vi "test Digital Pattern Output.vi"(8 "error in (no error)":errorcluster, 11 "TestCase in":refnum<class "Engine Simulation IO System Tests.lvclass">) -> (0 "error out":errorcluster, 3 "TestCase out":refnum<class "Engine Simulation IO System Tests.lvclass">)   [LabVIEW 2015, in "Engine Simulation IO System Tests.lvclass"]
uses:
  Engine Simulation IO System Tests.lvclass
  Engine Simulation IO System Tests.lvclass/Engine Simulation IO System Tests.ctl
  <vilib>/NI/LVFPGA Adv Session Resources/OpenByNameSubVI.vi
  <vilib>/NI Veristand/Execution/Workspace/NI VeriStand - Set Single Channel Value.vi
  <vilib>/rvi/interface/common/dynamic/niFpgaEscapeDelimiterAndNull.vi
  <vilib>/Utility/error.llb/Error Cluster From Error Code.vi
  <vilib>/rvi/errors/niLvFpgaAdjustHostInterfaceError.vi
  <vilib>/FPGAPlugInAG/Dynamic/niLvFpga_Close_Dynamic.vi
  <vilib>/NI/LVFPGA Adv Session Resources/OpenByName.xnode
  <vilib>/rvi/interface/nirviReadWriteControl/nirviReadWriteControl.xnode
  <vilib>/rvi/interface/nirviCloseFPGA/nirviCloseFPGA.xnode
  <vilib>/addons/_JKI Toolkits/VI Tester/TestCase.llb/TestCase.lvclass
  <vilib>/NI VeriStand/Execution/Workspace/NI_VS Workspace ExecutionAPI.lvlib
  System Explorer/Digital Pattern Find Events Enum.ctl
  System Explorer/Engine Simulation Toolkit System Explorer.lvlib
  NiFpgaLv.dll
  <vilib>/rvi/interface/Simulation/niFpgaSimulationCallBeginRW.vi
  System Explorer/Digital Pattern Add Pulse.ctl
  System Explorer/Digital Pattern Remove Edge.ctl
  System Explorer/Digital Pattern Base.ctl
  System Explorer/Digital Pattern.ctl
  <vilib>/NI/LVFPGA Adv Session Resources/LVFPGAAdvSessionResources.lvlib
panel:
  out "Values":T1(array[cluster])
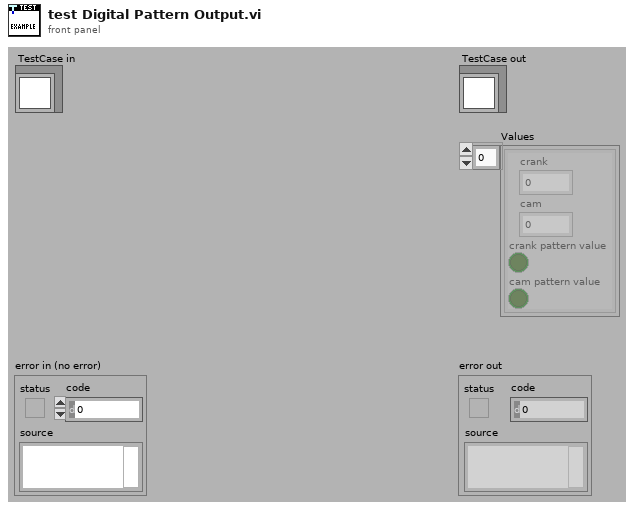
[diagram p1: front panel]
types:
  T1 = cluster{"crank":u16, "cam":u16, "crank pattern value":bool, "cam pattern value":bool}[]
  T2 = typedef "Engine Simulation Toolkit System Explorer.lvlib/Digital Pattern.ctl" = cluster{"Name":string, "Base":T3, "Remove":T4[], "Add":T5[], "FPGA Resource":string}
  T3 = typedef "Engine Simulation Toolkit System Explorer.lvlib/Digital Pattern Base.ctl" = cluster{"Length":dbl, "Teeth":u16, "Width":dbl, "Offset":dbl}
  T4 = typedef "Engine Simulation Toolkit System Explorer.lvlib/Digital Pattern Remove Edge.ctl" = cluster{"Tooth":u16, "Edge":bool}
  T5 = typedef "Engine Simulation Toolkit System Explorer.lvlib/Digital Pattern Add Pulse.ctl" = cluster{"Tooth":u16, "Offset":dbl, "Width":dbl}
  T6 = typedef "Engine Simulation Toolkit System Explorer.lvlib/Digital Pattern Find Events Enum.ctl" = enum16{"Rising Edge", "Falling Edge", "Any Edge", "Center Tooth", "Center Gap"}
  T7 = cluster{"Name":string, "Depth":u32, "Write? (Deprecated:Use Implementation)":bool, "Physical Channel":u32, "Base Address":u32, "Data Width":u32, "Data Type":enum32{"Boolean", "I8", "I16", "I32", "I64", "U8", "U16", "U32", "U64", "FXP", "CustomControl", "SGL"}, "FXP Properties":variant, "Write Window Address":u32, "Implementation":enum16{"niFpgaTargetToHost", "niFpgaHostToTarget", "niFpgaPeerToPeerWriter", "niFpgaPeerToPeerReader", "niCoreTargetToHost", "niCoreHostToTarget"}, "Control Set":u32}[]
  T8 = cluster{"Name":string, "type":variant, "indicator?":bool}[]
  T9 = typedef "NI_VS Workspace ExecutionAPI.lvlib/WorkspaceAPI.ctl" = refnum<k24>
  T10 = typedef "Engine Simulation Toolkit System Explorer.lvlib/Digital Pattern Expanded.ctl" = cluster{"X":dbl[], "Y":dbl[]}
  T11 = cluster{"crank":u16, "cam":u16, "crank pattern value":bool, "cam pattern value":bool}
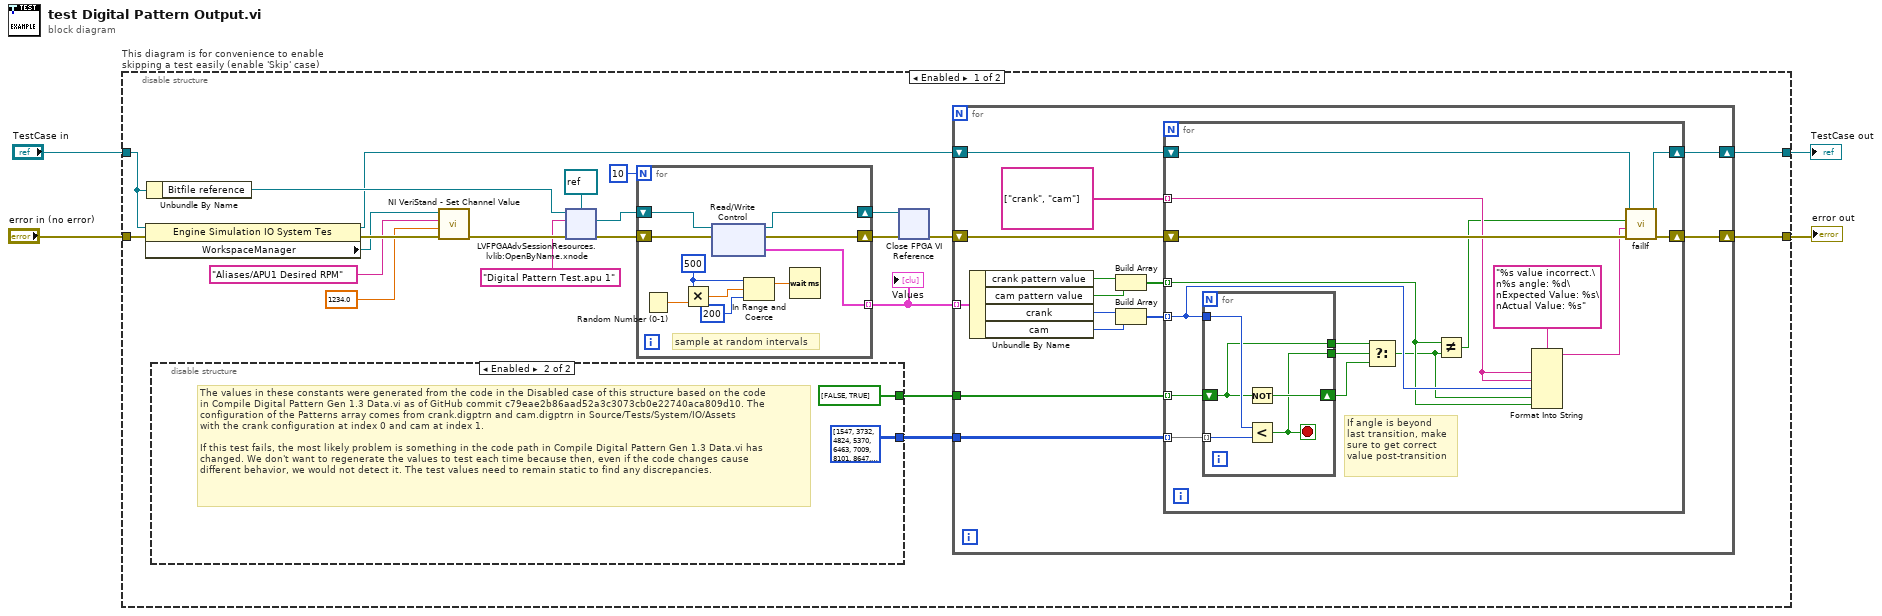
[diagram p0: block diagram]
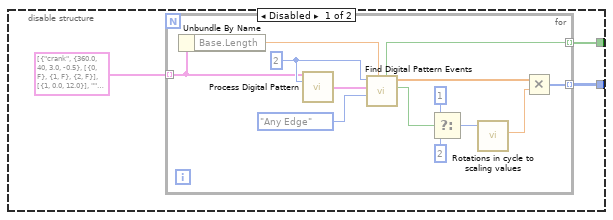
[diagram p2: hidden frame]
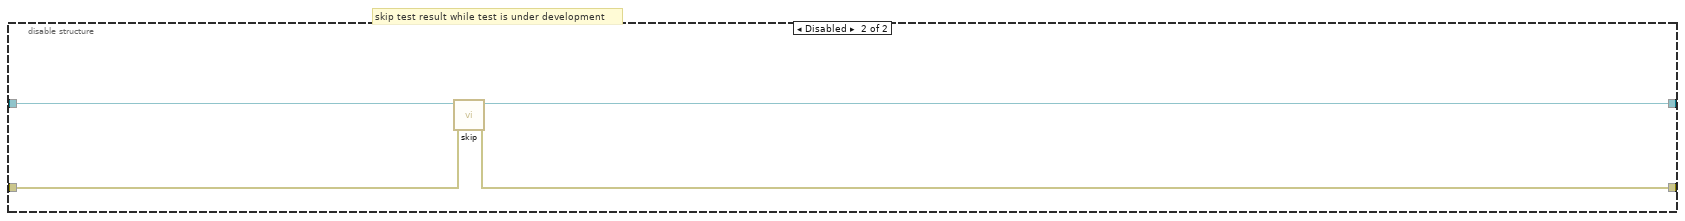
[diagram p3: hidden frame]
diagram:
  n1 = disable-structure "This diagram is for convenience to enable skipping a test easily (enable 'Skip' case)" shown="Enabled" {
    disable-tunnel: "TestCase in" -> [w9 w106]
    disable-tunnel: [w8 w104] -> w1
    disable-tunnel: [w5 w105] -> w3
    disable-tunnel: "error in (no error)" -> [w26 w103]
    frame Enabled {
      n2 = property class="Engine Simulation IO System Tes"(reference=w9, error in=w26) -> (reference out=w7:refnum<class "Engine Simulation IO System Tests.lvclass">, error out=w25:errorcluster, "WorkspaceManager"=w24:T9)
      n3 = Unbundle By Name(w9) -> ("Bitfile reference"=w20:refnum<k20>)
      n4 = disable-structure shown="Enabled" {
        disable-tunnel: [w29 bool[] [FALSE, TRUE] ("First Falling")] -> w11
        disable-tunnel: [w28 u16[][] [[1547, 3732, 4824, 5370, 6463, 7009, 8101, 8647, 9739, 10286, 11378, 11924, 13016, 13562, 14655, 15201, 16293, 16839, 17931, 18478, 19570, 20116, 21208, 21754, 22847, 23393, 24485, 25031, 26123, 26670, 27762, 28308, 29400, 29946, 31039, 31585, 32677, 33223, 34315, 34862, 35954, 36500, 37592, 38138, 39231, 39777, 40869, 41415, 42507, 43054, 44146, 44692, 45784, 46330, 47423, 47969, 49061, 49607, 50699, 51246, 52338, 52884, 53976, 54522, 55615, 56161, 57253, 57799, 58891, 59438, 60530, 61076, 62168, 62714, 63807, 64353], [4506, 13062, 17613, 26169, 30720, 39276, 43827, 52383, 56934, 65490, 0, 0, 0, 0, 0, 0, 0, 0, 0, 0, 0, 0, 0, 0, 0, 0, 0, 0, 0, 0, 0, 0, 0, 0, 0, 0, 0, 0, 0, 0, 0, 0, 0, 0, 0, 0, 0, 0, 0, 0, 0, 0, 0, 0, 0, 0, 0, 0, 0, 0, 0, 0, 0, 0, 0, 0, 0, 0, 0, 0, 0, 0, 0, 0, 0, 0]] ("Position LUT")] -> w10
        frame Disabled {
          n5 = for {
            tunnel: T2[] [{"Name"="crank", "Base"={"Length"=360.0, "Teeth"=40, "Width"=3.0, "Offset"=-0.5}, "Remove"=[{"Tooth"=0, "Edge"=FALSE}, {"Tooth"=1, "Edge"=FALSE}, {"Tooth"=2, "Edge"=FALSE}], "Add"=[{"Tooth"=1, "Offset"=0.0, "Width"=12.0}], "FPGA Resource"=""}, {"Name"="cam", "Base"={"Length"=720.0, "Teeth"=5, "Width"=50.0, "Offset"=-0.5}, "Remove"=[], "Add"=[], "FPGA Resource"=""}] ("Patterns") -> [w39] mode=indexing
            tunnel: [w36] -> w28 mode=indexing
            tunnel: [w30] -> w29 mode=indexing
            w41 = u16 2 ("Rotations")
            n6 = Unbundle By Name(w39) -> ("Base.Length"=w31:dbl)
            n7 = call "Process Digital Pattern.vi"("EPT Pattern"=w39, "Rotations"=w41) -> ("Final"=w42:T10)  [unwired: 7 in, 6 out]
            n8 = call "Find Digital Pattern Events.vi"("Base.length"=w31, "Event"=Digital_Pattern_Find_Events_Enum."Any Edge", "Pattern"=w42, "Rotations"=w41) -> ("crank angle"=w33:bool, "Locations"=w38:dbl[], "first falling"=w30:bool)  [unwired: 5 in]
            n9 = Select(t=u16 1 ("Rotations"), s=w33, f=u16 2 ("Rotations")) -> (s? t:f=w32:u16)
            n10 = call "Rotations in cycle to scaling values.vi"("rotations in a cycle"=w32) -> ("angle to u16 scale factor"=w37:dbl)  [unwired: 8 in, 2 out]
            n11 = Multiply(x=w38, y=w37) -> (x*y=w36:u16[])
          }
        }
        frame Enabled {
          # "The values in these constants were generated from the code in the Disabled case of this structure based on the code\nin Compile Digital Pattern Gen 1.3 Data.vi as of GitHub commit c79eae2b86aad52a3c3073cb0e22740aca809d10. The\nconfiguration of the Patterns array comes from crank.digptrn and cam.digptrn in Source/Tests/System/IO/Assets\nwith the crank configuration at index 0 and cam at index 1.\n\nIf this test fails, the most likely problem is something in the code path in Compile Digital Pattern Gen 1.3 Data.vi has\nchanged. We don't want to regenerate the values to test each time because then, even if the code changes cause\ndifferent behavior, we would not detect it. The test values need to remain static to find any discrepancies."
        }
      }
      n12 = call-poly <vilib>:"NI VeriStand - Set Channel Value.vi"("error in (no error)"=w25, "Value"=1234.0, "Channel"="Aliases/APU1 Desired RPM", "WorkspaceManager in"=w24) -> ("error out"=w21:errorcluster)  [unwired: 6 in, 1 out]
      n13 = xnode "LVFPGAAdvSessionResources.lvlib:OpenByName.xnode"("FPGA VI Reference in"=w20, "Resource name in"="Digital Pattern Test.apu 1", "Single resource reference type in"=refnum<k20> refnum, "Error in"=w21) -> ("Single resource reference out"=w16:refnum<k20>, "Error out"=w17:errorcluster)  [unwired: 1 out]
      n14 = for {
        N: 10 -> [_]
        shift-right: [w88] -> w14
        shift-left: w17 -> [w89]
        shift-right: [w86] -> w13
        shift-left: w16 -> [w87]
        tunnel: [w85] -> w12 mode=indexing
        w83 = u32 500 ("milliseconds to wait")
        # "sample at random intervals"
        n15 = Random Number (0-1)() -> (number: 0 to 1=w84:dbl)
        n16 = Multiply(x=w83, y=w84) -> (x*y=w82:dbl)
        n17 = xnode "Read/Write Control"("FPGA VI Reference In"=w87, "error in"=w89) -> ("FPGA VI Reference Out"=w86:refnum<k20>, "error out"=w88:errorcluster, "Value"=w85:T11)
        n18 = In Range and Coerce(upper limit=w83, x=w82, lower limit=u32 200 ("milliseconds to wait")) -> (coerced(x)=w80:dbl)  [unwired: 1 out]
        n19 = Wait (ms)(milliseconds to wait=w80) -> ()  [unwired: 1 out]
      }
      "Values" <- w12
      n20 = xnode "Close FPGA VI Reference"("FPGA VI Reference In"=w13, "error in"=w14) -> ("error out"=w6:errorcluster)
      n21 = for {
        tunnel: w12 -> [w58] mode=indexing
        tunnel: w11 -> [w57]
        tunnel: w10 -> [w56]
        shift-right: [w51] -> w8
        shift-left: w7 -> [w52]
        shift-right: [w49] -> w5
        shift-left: w6 -> [w50]
        n22 = Unbundle By Name(w58) -> ("crank pattern value"=w48:bool, "cam pattern value"=w47:bool, "crank"=w55:u16, "cam"=w54:u16)
        n23 = Build Array(w48, w47) -> (w46:bool[])
        n24 = Build Array(w55, w54) -> (w53:u16[])
        n25 = for {
          tunnel: w57 -> [w73] mode=indexing
          tunnel: w56 -> [w74] mode=indexing
          tunnel: w53 -> [w64] mode=indexing
          shift-right: [w70] -> w51
          shift-left: w52 -> [w69]
          shift-right: [w71] -> w49
          shift-left: w50 -> [w72]
          tunnel: w46 -> [w63] mode=indexing
          tunnel: string[] ["crank", "cam"] -> [w67] mode=indexing
          # "If angle is beyond\nlast transition, make\nsure to get correct\nvalue post-transition"
          n26 = for {
            tunnel: w74 -> [w78] mode=indexing
            tunnel: w64 -> [w79]
            shift-right: [w77] -> w60
            shift-left: w73 -> [w76]
            tunnel: [w76] -> w61
            tunnel: [w75] -> w62
            stop <- w75 stop-if-true
            n27 = Not(x=w76) -> (.not. x?=w77:bool)
            n28 = Less?(x=w79, y=w78) -> (x < y?=w75:bool)
          }
          n29 = Select(t=w61, s=w62, f=w60) -> (s? t:f=w59:bool)
          n30 = Not Equal?(x=w63, y=w59) -> (x != y?=w66:bool)
          n31 = Format Into String(format string="%s value incorrect.\n%s angle: %d\nExpected Value: %s\nActual Value: %s", w67, w67, w64, w59, w63) -> (resulting string=w65:string)  [unwired: 2 in, 1 out]
          n32 = call-dynamic "failIf.vi"("error in (no error)"=w72, "message (\"\")"=w65, "fail"=w66, "TestCase in"=w69) -> ("error out"=w71:errorcluster, "TestCase out"=w70:refnum<class "Engine Simulation IO System Tests.lvclass">)  [unwired: 6 in]
        }
      }
    }
    frame Disabled {
      # "skip test result while test is under development"
      n33 = call <vilib>:"skip.vi"("error in (no error)"=w103, "TestCase in"=w106) -> ("error out"=w105:errorcluster, "TestCase out"=w104:refnum<class "Engine Simulation IO System Tests.lvclass">)  [unwired: 8 in]
    }
  }
  "error out" <- w3
  "TestCase out" <- w1
